vi "LVClass_Camera get image.vi"(0 "Camera in":refnum<class "Camera.lvclass">, 5 "Image":refnum<class "Image.lvclass">, 7 "Image RAW":refnum<class "Image.lvclass">, 9 "remove_background":bool=TRUE, 11 "error in (no error)":errorcluster) -> (4 "Camera out":refnum<class "Camera.lvclass">, 6 "Image (dup)":refnum<class "Image.lvclass">, 8 "Image (dup) RAW":refnum<class "Image.lvclass">, 15 "error out":errorcluster)   [LabVIEW 2020, in "Camera.lvclass"]
doc: "Retrieve last captured image. see Imop_Camera_AsyncImageReady.\n\n--------------------------------------------------------------------------------\n\n<B>CameraIn </B> : Camera object.\n<B>CameraOut </B> : Camera object.\n<B>Image </B> : Captured image with (optionnally) background removed.\n<B>remove_background </B> : Boolean which indicates if background should be substracted.\n<B>RawImage </B> : Captured image without any post-processing applied.\n<B>ErrorIn </B> : Error\n<B>ErrorOut </B> : Error\n\n--------------------------------------------------------------------------------"
uses:
  Camera.lvclass
  Image.lvclass
  Camera.lvclass/Camera.ctl
  CameraAcquisitionState.ctl
  LVClass_Image read Image Compat ptr.vi
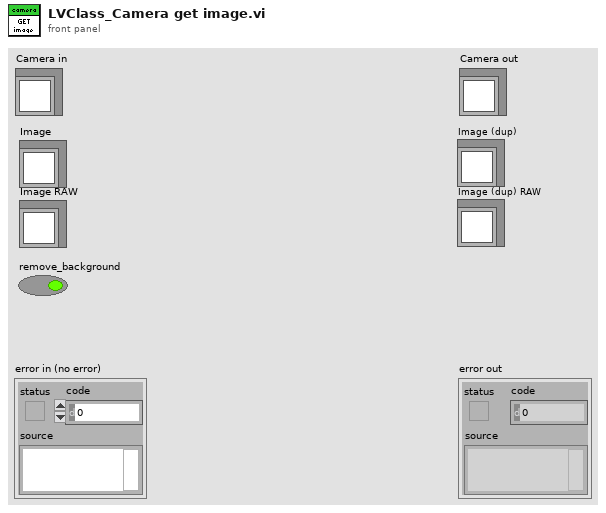
[diagram p1: front panel]
types:
  T1 = typedef "CameraAcquisitionState.ctl" = enum16{"Stop", "Live"}
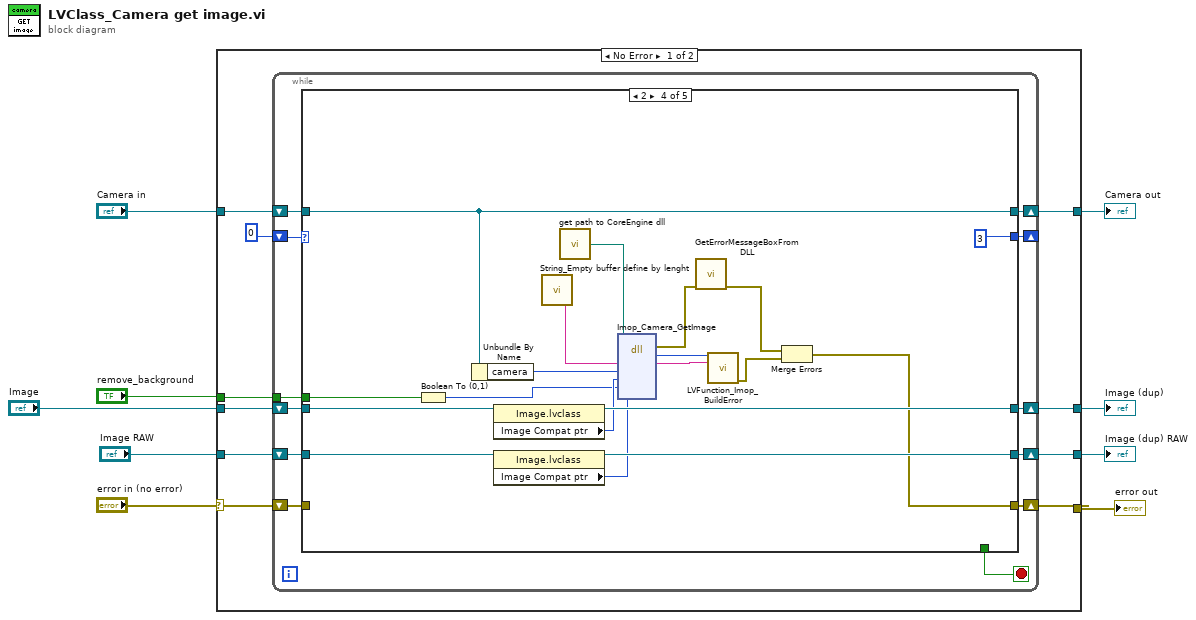
[diagram p0: block diagram]
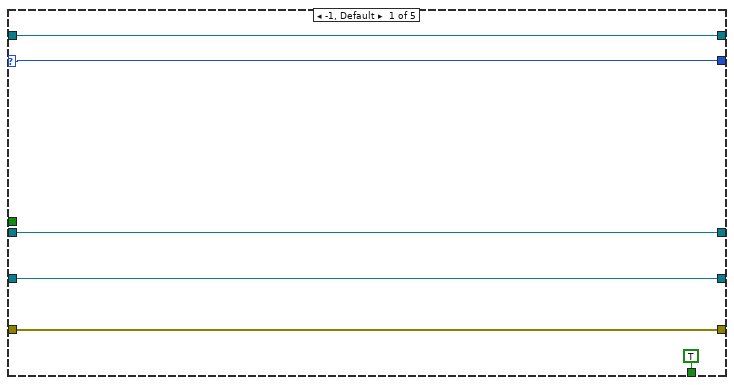
[diagram p2: hidden frame]
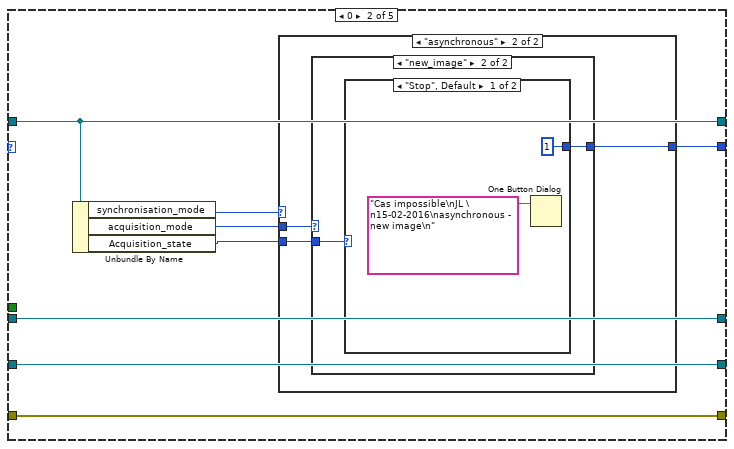
[diagram p3: hidden frame]
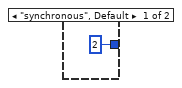
[diagram p4: hidden frame]
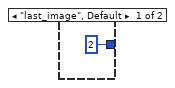
[diagram p5: hidden frame]
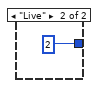
[diagram p6: hidden frame]
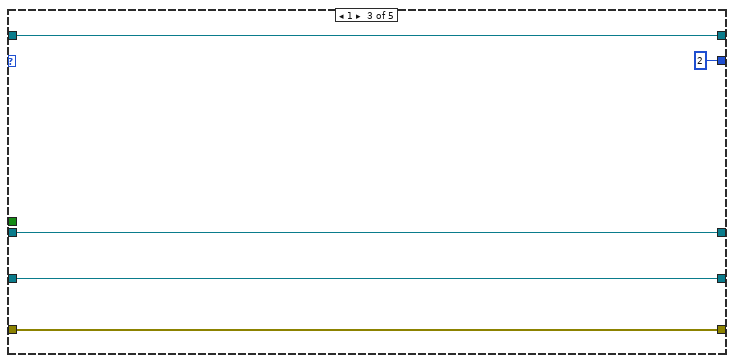
[diagram p7: hidden frame]
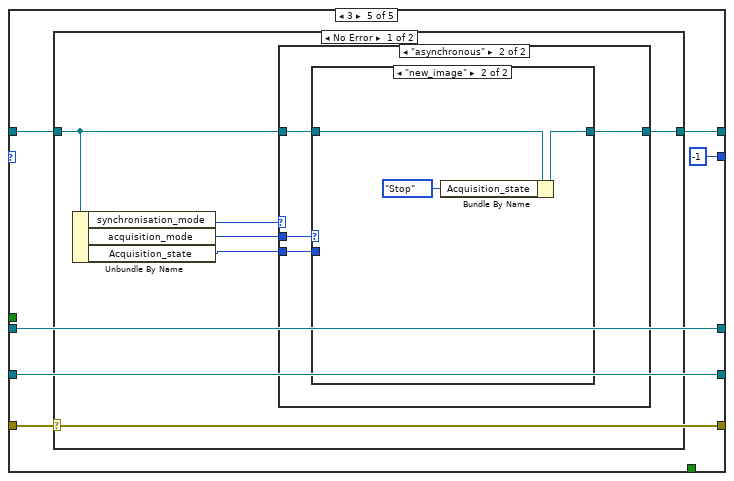
[diagram p8: hidden frame]
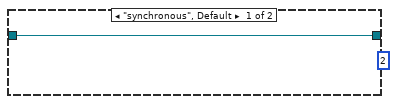
[diagram p9: hidden frame]
diagram:
  n1 = case shown="No Error" "error in (no error)" {
    selector: "error in (no error)" -> [w12 w104]
    tunnel: [w14 w104] -> w8
    tunnel: [w10 w103] -> w6
    tunnel: "Camera in" -> [w11 w103]
    tunnel: [w18 w102] -> w5
    tunnel: "Image" -> [w19 w102]
    tunnel: "Image RAW" -> [w17 w101]
    tunnel: [w16 w101] -> w2
    tunnel: "remove_background" -> [w15 _]
    frame No Error {
      n2 = while {
        tunnel: w15 -> [w27]
        shift-right: [w23] -> w10
        shift-left: w11 -> [w25]
        shift-right: [w30] -> w18
        shift-left: w19 -> [w31]
        shift-right: [w28] -> w16
        shift-left: w17 -> [w29]
        shift-right: [w26] -> w14
        shift-left: w12 -> [w22]
        shift-right: [w21] -> _
        shift-left: 0 -> [w24]
        stop <- w20 stop-if-true
        n3 = case shown="2" w24 {
          selector: w24 -> [w33 _ _ _ _]
          tunnel: w31 -> [w35 w39 w60 w79 w85]
          tunnel: [w35 w39 w60 w78 w85] -> w30
          tunnel: w29 -> [w34 w38 w59 w77 w84]
          tunnel: [w34 w38 w59 w76 w84] -> w28
          tunnel: w27 -> [_ _ _ w75 _]
          tunnel: [w37 w45 w56 w74 w80] -> w26
          tunnel: w25 -> [w36 w44 w57 w73 w82]
          tunnel: [w36 w44 w57 w73 w83] -> w23
          tunnel: w22 -> [w37 w45 w56 _ w80]
          tunnel: [w33 w40 2 3 -1] -> w21
          tunnel: [TRUE _ _ _ _] -> w20
          frame -1, Default {
          }
          frame 0 {
            n4 = Unbundle By Name(w44) -> ("synchronisation_mode"=w43:enum16{"synchronous", "asynchronous"}, "acquisition_mode"=w42:enum16{"last_image", "new_image"}, "Acquisition_state"=w41:T1)
            n5 = case shown="\"asynchronous\"" w43 {
              tunnel: w42 -> [_ w49]
              tunnel: w41 -> [_ w48]
              tunnel: [2 w47] -> w40
              frame "synchronous", Default {
              }
              frame "asynchronous" {
                n6 = case shown="\"new_image\"" w49 {
                  tunnel: w48 -> [_ w52]
                  tunnel: [2 w51] -> w47
                  frame "last_image", Default {
                  }
                  frame "new_image" {
                    n7 = case shown="\"Stop\", Default" w52 {
                      tunnel: [1 2] -> w51
                      frame "Stop", Default {
                        n8 = One Button Dialog(message="Cas impossible\nJL \n15-02-2016\nasynchronous - new image\n") -> ()  [unwired: 1 in, 1 out]
                      }
                      frame "Live" {
                      }
                    }
                  }
                }
              }
            }
          }
          frame 1 {
          }
          frame 2 {
            n9 = Boolean To (0,1)(Boolean=w75) -> (0, 1=w63:i16)
            n10 = Unbundle By Name(w73) -> ("camera"=w68:i32)
            n11 = property class="Image.lvclass"(reference=w79) -> (reference out=w78:refnum<class "Image.lvclass">, "Image Compat ptr"=w66:i32)  [unwired: 1 in, 1 out]
            n12 = property class="Image.lvclass"(reference=w77) -> (reference out=w76:refnum<class "Image.lvclass">, "Image Compat ptr"=w64:i32)  [unwired: 1 in, 1 out]
            n13 = call "String_Empty buffer define by lenght.vi"() -> ("Empty buffer"=w71:string)  [unwired: 1 in]
            n14 = call "get path to CoreEngine dll.vi"() -> ("path to c_interface_vc100.dll"=w67:path)  [unwired: 12 in, 3 out]
            n15 = dll-call lib="D:/soft/HASO_v3/SVN_trunk/ImOpCoreEngine4_LV2011/DLLs/c_interface_vc100.dll" fn="Imop_Camera_GetImage"(path in=w67, "message"=w71, "camera"=w68, "HASO_image"=w66, "remove background"=w63, "RAW HASO_image"=w64) -> (error out=w65:errorcluster, "return type"=w70:i32, "message"=w69:string)  [unwired: 6 in, 1 out]
            n16 = call "GetErrorMessageBoxFromDLL.vi"("error IN"=w65) -> ("error OUT"=w62:errorcluster)  [unwired: 10 in]
            n17 = call "LVFunction_Imop_BuildError.vi"("code"=w70, "String to Prepend to source (\"\")"=w69) -> ("error out"=w61:errorcluster)  [unwired: 13 in]
            n18 = Merge Errors(w62, w61) -> (w74:errorcluster)
          }
          frame 3 {
            n19 = case shown="No Error" w80 {
              tunnel: [w87 w100] -> w83
              tunnel: w82 -> [w86 w100]
              frame No Error {
                n20 = Unbundle By Name(w86) -> ("synchronisation_mode"=w90:enum16{"synchronous", "asynchronous"}, "acquisition_mode"=w89:enum16{"last_image", "new_image"}, "Acquisition_state"=w88:T1)
                n21 = case shown="\"asynchronous\"" w90 {
                  tunnel: w89 -> [_ w95]
                  tunnel: w88 -> [_ w94]
                  tunnel: [w91 w93] -> w87
                  tunnel: w86 -> [w91 w92]
                  frame "synchronous", Default {
                    (unwired) 2
                  }
                  frame "asynchronous" {
                    n22 = case shown="\"new_image\"" w95 {
                      tunnel: w94 -> [_ _]
                      tunnel: [w96 w97] -> w93
                      tunnel: w92 -> [w96 w98]
                      frame "last_image", Default {
                      }
                      frame "new_image" {
                        n23 = Bundle By Name(cluster=w98, "Acquisition_state"=CameraAcquisitionState."Stop") -> (w97:refnum<class "Camera.lvclass">)
                      }
                    }
                  }
                }
              }
              frame Error {
              }
            }
          }
        }
      }
    }
    frame Error {
    }
  }
  "error out" <- w8
  "Camera out" <- w6
  "Image (dup)" <- w5
  "Image (dup) RAW" <- w2
